vi "Simulate Sawtooth Signal.vi"(8 "error in (no error)":errorcluster) -> (0 "error out":errorcluster, 3 "Sawtooth with Uniform Noise":dynamicdata(graph))   [LabVIEW 2023, in "Scope Simulated CFGs.lvlib" / "Fetch Waveforms CFG.lvclass"]
uses:
  Fetch Waveforms CFG.lvclass
  Fetch Waveforms CFG.lvclass/Fetch Waveforms CFG.ctl
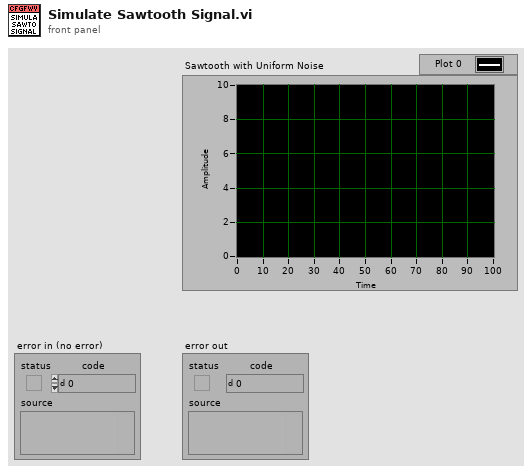
[diagram p1: front panel]
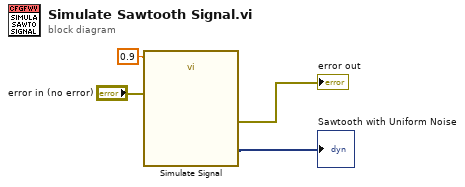
[diagram p0: block diagram]
diagram:
  n1 = call "Simulate Signal"("Offset"=0.9, "error in (no error)"="error in (no error)") -> ("Sawtooth with Uniform Noise"=→"Sawtooth with Uniform Noise":dynamicdata, "error out"=→"error out":errorcluster)  [unwired: 12 in]
